vi "PI Format Table Display.vi"(6 "Measurements":refnum<vi>, 8 "error in (no error)":errorcluster, 11 "Results":T1={"Measurement Cycles"=0, "Response"="", "Measurement"={"sxFieldId"="", "sValue"="", "nDataType"=enum."Scalar", "sUnits"="", "sDisplayName"=""}, "Limit"={"Limits On"=TRUE, "Limits"=[]}, "Status Array"=[]}) -> (0 "error out":errorcluster, 1 "Incomplete?":bool, 2 "All PASS?":bool, 3 "Strings to Display":string[][](array[string]), 4 "Message":string, 5 "Results Out":T1={"Measurement Cycles"=0, "Response"="", "Measurement"={"sxFieldId"="", "sValue"="", "nDataType"=enum."Scalar", "sUnits"="", "sDisplayName"=""}, "Limit"={"Limits On"=TRUE, "Limits"=[]}, "Status Array"=[]})   [LabVIEW 2011]
uses:
  TypeDefs/PI Results.ctl
  TypeDefs/PI Measurement Cluster.ctl
  TypeDefs/PI Limit Parameters.ctl
  TypeDefs/PI Limit Definition.ctl
  TypeDefs/PI Limit Comparison.ctl
  Test Status.ctl
panel:
  in  "Colors":cluster{"Pass":u32, "Fail":u32, "Nop":u32}={"Pass"=6618880, "Fail"=16711680, "Nop"=16777226}
  out "PF":string[](array[string])
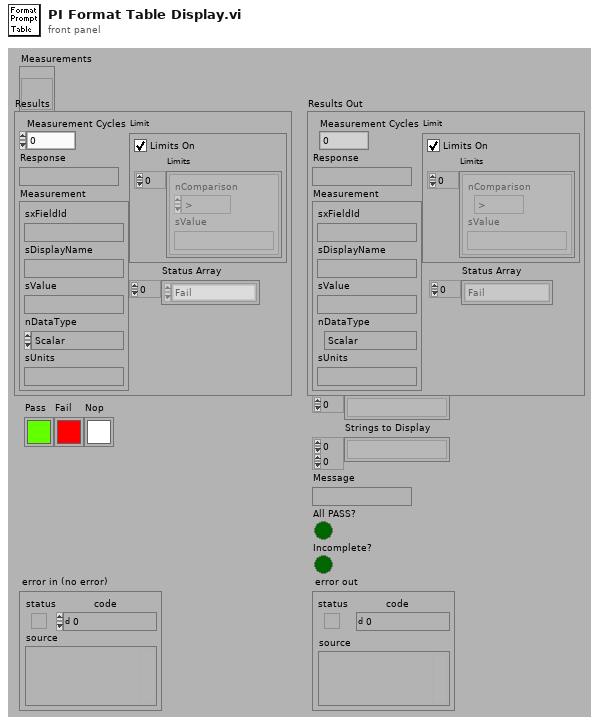
[diagram p1: front panel]
types:
  T1 = typedef "PI Results.ctl" = cluster{"Measurement Cycles":i32, "Response":string, "Measurement":T2, "Limit":T3, "Status Array":enum16{"Fail", "Pass", "Abort", "Error", "Done", "Pass by Sample", "Fail by Sample", "Pass Override", "Fail Override", "Not Tested"}[]}
  T2 = typedef "PI Measurement Cluster.ctl" = cluster{"sxFieldId":string, "sValue":string, "nDataType":enum16{"Scalar", "Enumeration"}, "sUnits":string, "sDisplayName":string}
  T3 = typedef "PI Limit Parameters.ctl" = cluster{"Limits On":bool, "Limits":T4[]}
  T4 = typedef "PI Limit Definition.ctl" = cluster{"nComparison":T5, "sValue":string}
  T5 = typedef "PI Limit Comparison.ctl" = enum16{">", ">=", "<", "<=", "<>", "="}
  T6 = typedef "Test Status.ctl" = enum16{"Fail", "Pass", "Abort", "Error", "Done", "Pass by Sample", "Fail by Sample", "Pass Override", "Fail Override", "Not Tested"}
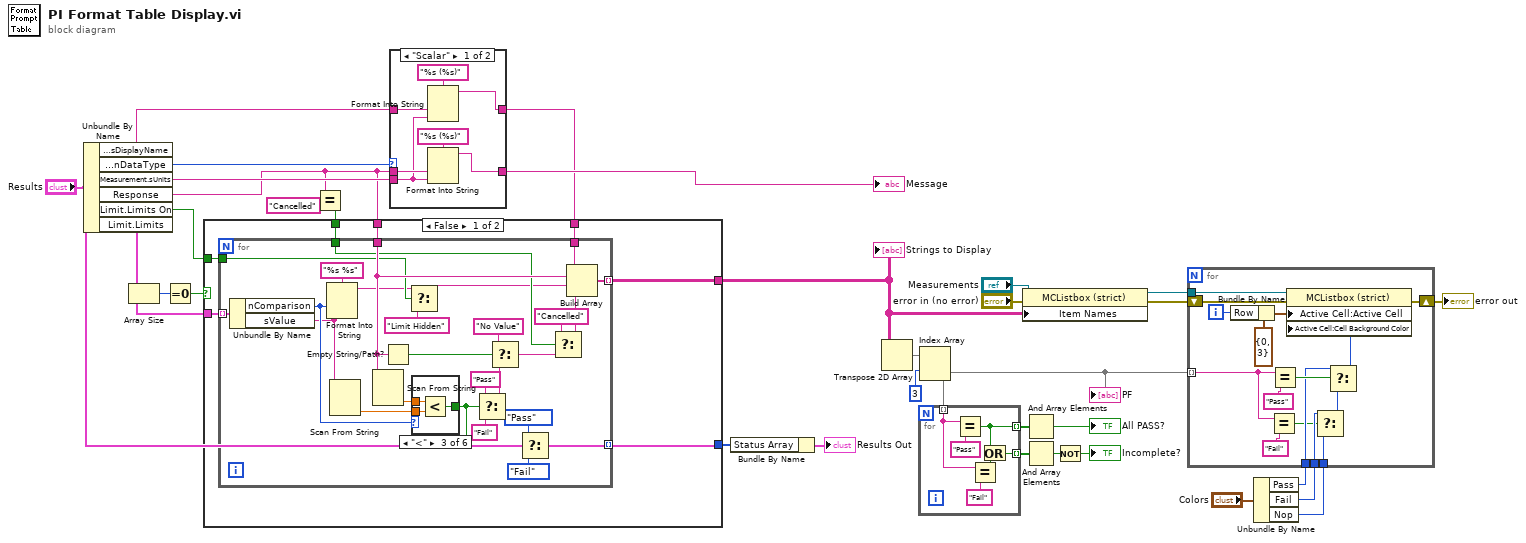
[diagram p0: block diagram]
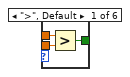
[diagram p3: hidden frame]
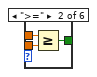
[diagram p4: hidden frame]
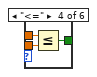
[diagram p5: hidden frame]
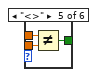
[diagram p6: hidden frame]
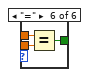
[diagram p7: hidden frame]
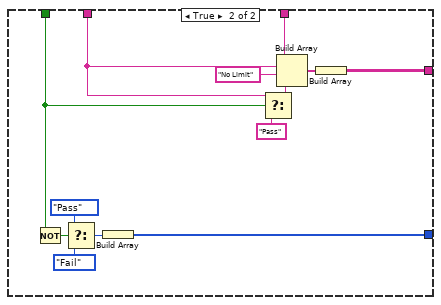
[diagram p8: hidden frame]
diagram:
  n1 = Unbundle By Name("Results") -> ("Measurement.sDisplayName"=w4:string, "Measurement.nDataType"=w6:enum16{"Scalar", "Enumeration"}, "Measurement.sUnits"=w5:string, "Response"=w2:string, "Limit.Limits On"=w1:bool, "Limit.Limits"=w15:T4[])
  n2 = Array Size(array=w15) -> (size(s)=w21:i32)
  n3 = Equal To 0?(x=w21) -> (x = 0?=w20:bool)
  n4 = Equal?(x=w2, y="Cancelled") -> (x = y?=w18:bool)
  n5 = case shown="\"Scalar\"" w6 {
    tunnel: w2 -> [w39 w42]
    tunnel: w5 -> [w36 _]
    tunnel: [w38 w42] -> w14
    tunnel: w4 -> [w35 w41]
    tunnel: [w34 w41] -> w3
    frame "Scalar" {
      n6 = Format Into String(format string="%s (%s)", w35, w36) -> (resulting string=w34:string)  [unwired: 2 in, 1 out]
      n7 = Format Into String(format string="%s (%s)", w39, w36) -> (resulting string=w38:string)  [unwired: 2 in, 1 out]
    }
    frame "Enumeration" {
    }
  }
  "Message" <- w14
  n8 = case shown="False" w20 {
    tunnel: w15 -> [w49 _]
    tunnel: w3 -> [w48 w106]
    tunnel: w2 -> [w47 w101]
    tunnel: [w46 w103] -> w16
    tunnel: w18 -> [w45 w99]
    tunnel: [w44 w95] -> w17
    tunnel: w1 -> [w43 _]
    frame False {
      n9 = for {
        tunnel: w49 -> [w75] mode=indexing
        tunnel: w48 -> [w74]
        tunnel: w47 -> [w65]
        tunnel: [w66] -> w46 mode=indexing
        tunnel: w45 -> [w54]
        tunnel: [w58] -> w44 mode=indexing
        tunnel: w43 -> [w53]
        n10 = Unbundle By Name(w75) -> ("nComparison"=w72:T5, "sValue"=w71:string)
        n11 = Format Into String(format string="%s %s", w72, w71) -> (resulting string=w52:string)  [unwired: 2 in, 1 out]
        n12 = Scan From String(input string=w71) -> (output 1=w70:dbl)  [unwired: 3 in, 4 out]
        n13 = Scan From String(input string=w65) -> (output 1=w69:dbl)  [unwired: 3 in, 4 out]
        n14 = Empty String/Path?(string/path=w65) -> (empty?=w64:bool)
        n15 = Select(t=w52, s=w53, f="Limit Hidden" ("format string")) -> (s? t:f=w51:string)
        n16 = case shown="\"<\"" w72 {
          tunnel: w70 -> [w77 w80 w83 w86 w89 w92]
          tunnel: w69 -> [w78 w81 w84 w87 w90 w93]
          tunnel: [w76 w79 w82 w85 w88 w91] -> w57
          frame ">", Default {
            n17 = Greater?(x=w78, y=w77) -> (0:w76:bool)
          }
          frame ">=" {
            n18 = Greater Or Equal?(x=w81, y=w80) -> (x >= y?=w79:bool)
          }
          frame "<" {
            n19 = Less?(x=w84, y=w83) -> (x < y?=w82:bool)
          }
          frame "<=" {
            n20 = Less Or Equal?(x=w87, y=w86) -> (x <= y?=w85:bool)
          }
          frame "<>" {
            n21 = Not Equal?(x=w90, y=w89) -> (x != y?=w88:bool)
          }
          frame "=" {
            n22 = Equal?(x=w93, y=w92) -> (x = y?=w91:bool)
          }
        }
        n23 = Select(t="Pass" ("format string"), s=w57, f="Fail" ("format string")) -> (s? t:f=w63:string)
        n24 = Select(t="No Value" ("format string"), s=w64, f=w63) -> (s? t:f=w60:string)
        n25 = Select(t=Test_Status."Pass" ("Test Status"), s=w57, f=Test_Status."Fail" ("Test Status")) -> (s? t:f=w58:T6)
        n26 = Select(t="Cancelled" ("format string"), s=w54, f=w60) -> (s? t:f=w59:string)
        n27 = Build Array(w74, w65, w51, w59) -> (w66:string[])
      }
    }
    frame True {
      n28 = Not(x=w99) -> (.not. x?=w96:bool)
      n29 = Select(t=Test_Status."Pass" ("Test Status"), s=w96, f=Test_Status."Fail" ("Test Status")) -> (s? t:f=w94:T6)
      n30 = Build Array(w94) -> (w95:T6[])
      n31 = Select(t=w101, s=w99, f="Pass") -> (s? t:f=w100:string)
      n32 = Build Array(w106, w101, "No Limit", w100) -> (w104:string[])
      n33 = Build Array(w104) -> (w103:string[][])
    }
  }
  "Strings to Display" <- w16
  n34 = Bundle By Name(cluster="Results", "Status Array"=w17) -> (→"Results Out":T1)
  n35 = Transpose 2D Array(2D array=w16) -> (transposed array=w32:string[][])
  n36 = Index Array(array=w32, index (row)=3) -> (element=w11:string[])  [unwired: 1 in]
  "PF" <- w11
  n37 = for {
    tunnel: [w109] -> w26 mode=indexing
    tunnel: w11 -> [w110] mode=indexing
    tunnel: [w107] -> w24 mode=indexing
    n38 = Equal?(x=w110, y="Pass") -> (x = y?=w109:bool)
    n39 = Equal?(x=w110, y="Fail") -> (x = y?=w108:bool)
    n40 = Or(x=w109, y=w108) -> (x .or. y?=w107:bool)
  }
  n41 = property class="MCListbox (strict)"(reference="Measurements", error in="error in (no error)", "Item Names"=w16) -> (reference out=w31:refnum<vi>, error out=w10:errorcluster)
  n42 = And Array Elements(Boolean array=w26) -> (logical AND=→"All PASS?":bool)
  n43 = And Array Elements(Boolean array=w24) -> (logical AND=w23:bool)
  n44 = Not(x=w23) -> (.not. x?=→"Incomplete?":bool)
  n45 = Unbundle By Name("Colors") -> ("Pass"=w29:u32, "Fail"=w28:u32, "Nop"=w27:u32)
  n46 = for {
    tunnel: w31 -> [w128]
    tunnel: w29 -> [w122]
    tunnel: w28 -> [w119]
    tunnel: w27 -> [w117]
    tunnel: w11 -> [w115] mode=indexing
    shift-right: [w113] -> w9
    shift-left: w10 -> [w114]
    i -> [w126]
    n47 = Bundle By Name(cluster=cluster{"Row":i32, "Column":i32} {"Row"=0, "Column"=3} ("Active Cell"), "Row"=w126) -> (w125:cluster{"Row":i32, "Column":i32})
    n48 = Equal?(x=w115, y="Fail") -> (x = y?=w116:bool)
    n49 = Equal?(x=w115, y="Pass") -> (x = y?=w123:bool)
    n50 = Select(t=w119, s=w116, f=w117) -> (s? t:f=w118:u32)
    n51 = Select(t=w122, s=w123, f=w118) -> (s? t:f=w121:u32)
    n52 = property class="MCListbox (strict)"(reference=w128, error in=w114, "Active Cell:Active Cell"=w125, "Active Cell:Cell Background Color"=w121) -> (error out=w113:errorcluster)  [unwired: 1 out]
  }
  "error out" <- w9
